vi "LogGitHash.vi"(8 "error in (no error)":errorcluster) -> (0 "error out":errorcluster)   [LabVIEW 2018, in "feGEM DataPacker.lvlib"]
uses:
  feGEM DataPacker.lvlib
  073cd073-7df5-4552-9782-90e5463131dd.vi
  dbafba9a-7b14-4d39-925e-628497f365c2.vi
  GitTools/GitCommitData.ctl
panel:
  out "Array":T1[](array[typedef])
  out ".git log paths":path[](array[path])
  out ".git hash paths":path[](array[path])
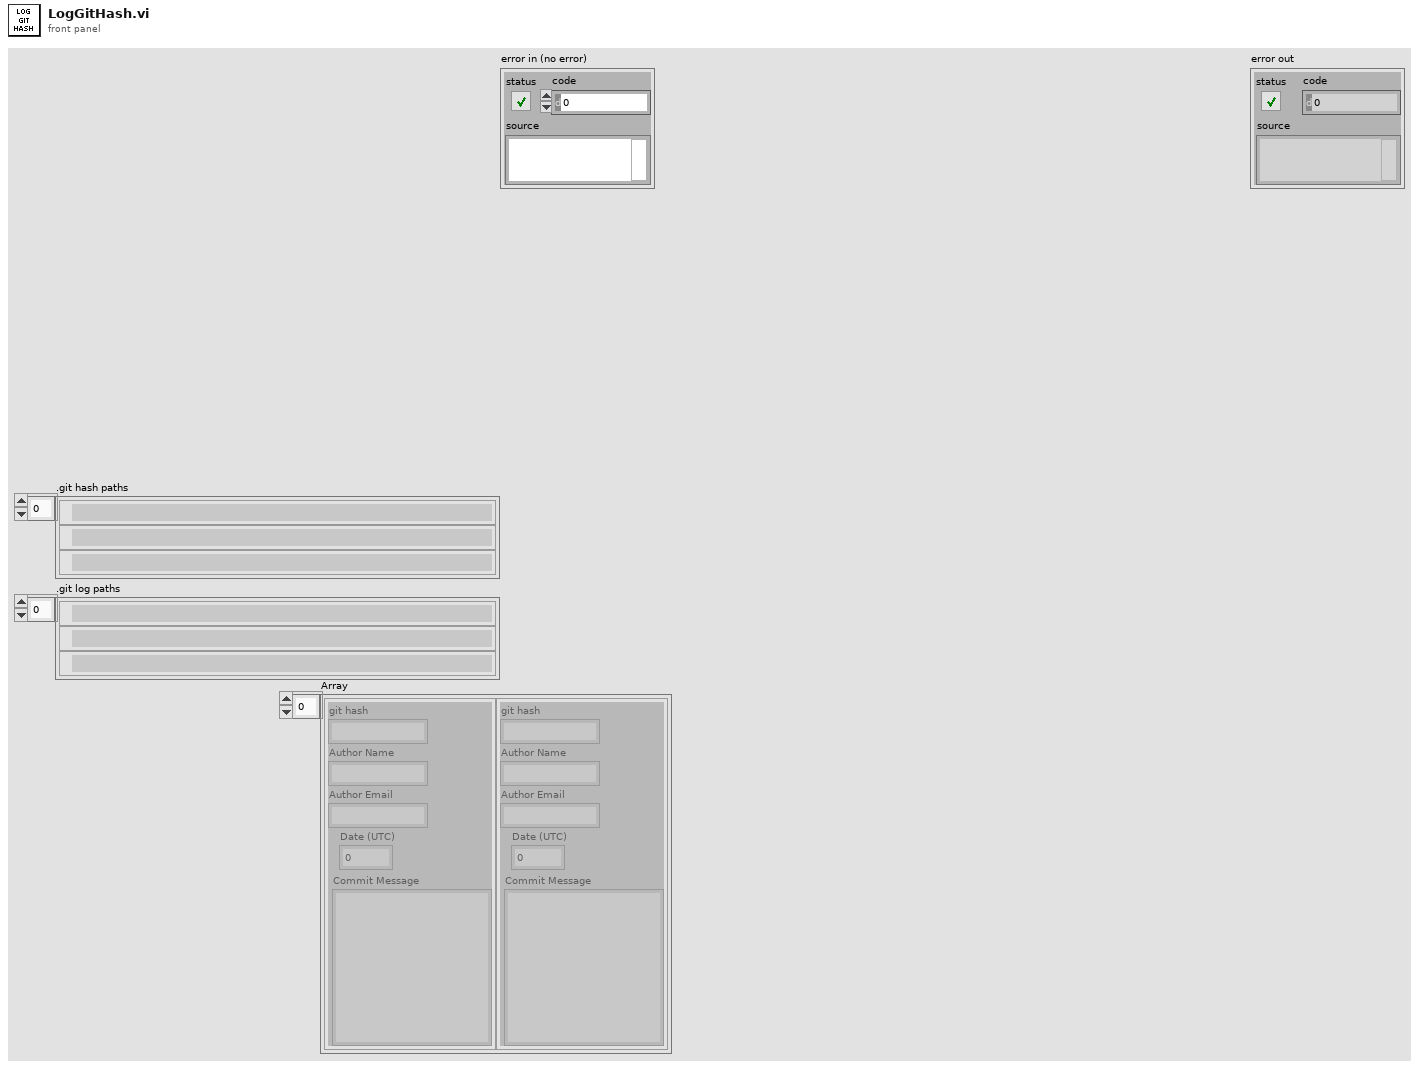
[diagram p1: front panel]
types:
  T1 = typedef "feGEM DataPacker.lvlib/GitCommitData.ctl" = cluster{"git hash":string, "Author Name":string, "Author Email":string, "Date (UTC)":i32, "Commit Message":string}
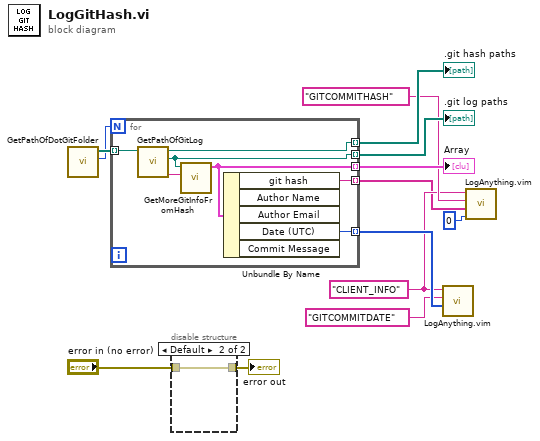
[diagram p0: block diagram]
diagram:
  w4 = "CLIENT_INFO" ("Category")
  n1 = call "GetPathOfDotGitFolder.vi"() -> ("Number of nested git modules"=w11:i32, ".git folder paths"=w12:path[])  [unwired: 10 in]
  n2 = for {
    N: w11 -> [_]
    tunnel: w12 -> [w19] mode=indexing
    tunnel: [w18] -> w10 mode=indexing
    tunnel: [w17] -> w9 mode=indexing
    tunnel: [w16] -> w8 mode=indexing
    tunnel: [w15] -> w5 mode=indexing
    tunnel: [w14] -> w2 mode=indexing
    n3 = call "GetPathOfGitLog.vi"("Path"=w19) -> ("git hash (version)"=w20:string, "git log file path"=w17:path, "git hash file path"=w18:path)  [unwired: 7 in, 1 out]
    n4 = call "GetMoreGitInfoFromHash.vi"("git hash"=w20, "git hash file path"=w17) -> ("git commit"=w16:T1)  [unwired: 8 in, 1 out]
    n5 = Unbundle By Name(w16) -> ("git hash"=w14:string, "Date (UTC)"=w15:i32)  [unwired: 3 out]
  }
  ".git hash paths" <- w10
  ".git log paths" <- w9
  "Array" <- w8
  n6 = disable-structure shown="Default" {
    disable-tunnel: "error in (no error)" -> [w21 w22]
    disable-tunnel: [w21 w22] -> w1
    frame condition #0 (active) {
    }
    frame condition #1 {
    }
  }
  "error out" <- w1
  n7 = call "LogAnything.vim"("Array"=w5, "Var Name"="GITCOMMITDATE", "Category"=w4) -> ()  [unwired: 4 in, 1 out]
  n8 = call "LogAnything.vim"("Period to update history plots (seconds)\nUnset (65535) = Use MIDAS default in ODB\n0 = Record but do not put in histories"=u16 0 ("Period to update history plots (seconds)\nUnset (65535) = Use MIDAS default in ODB\n0 = Record but do not put in histories"), "Array"=w2, "Var Name"="GITCOMMITHASH", "Category"=w4) -> ()  [unwired: 3 in, 1 out]
